vi "Header.vi"(8 "error in (no error)":errorcluster) -> (0 "error out":errorcluster, 3 "Headers":string)   [LabVIEW 2013]
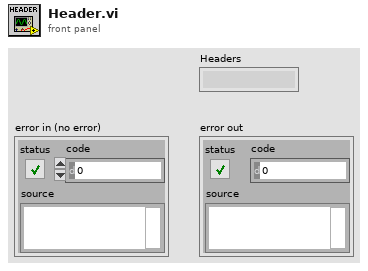
[diagram p1: front panel]
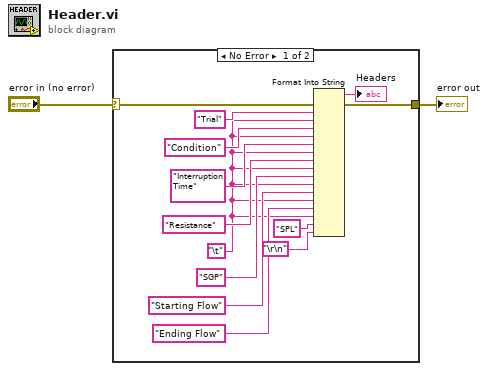
[diagram p0: block diagram]
diagram:
  n1 = case shown="No Error" "error in (no error)" {
    selector: "error in (no error)" -> [w13 w16]
    tunnel: [w14 w16] -> w2
    frame No Error {
      w5 = "\t"
      n2 = Format Into String(error in=w13, "Trial", w5, "Condition" ("input 3"), w5, "Interruption Time" ("format string"), w5, "Resistance" ("format string"), w5, "SGP" ("format string"), w5, "Starting Flow" ("input 11"), w5, "Ending Flow" ("input 13"), w5, "SPL" ("input 15"), "\r\n") -> (resulting string=→"Headers":string, error out=w14:errorcluster)  [unwired: 2 in]
    }
    frame Error {
    }
  }
  "error out" <- w2
